vi "autoshoot.vi"() -> ()   [LabVIEW 2012]
uses:
  <vilib>/Platform/TimedLoop/XDataNode/wakeup.ctl
  <vilib>/Platform/TimedLoop/XDataNode/XDNodeRunTimeDep.lvlib
  <vilib>/Platform/TimedLoop/XDataNode/nitl_modes.ctl
  <vilib>/Platform/TimedLoop/XDataNode/timing_clust.ctl
  <vilib>/platform/TimedLoop/XDataNode/XDataNode.xnode
  <vilib>/Rock Robotics/WPI/RobotDrive/WPI_RobotDriveArcadeDrive_Standard(NoSaturation).vi
  <vilib>/Rock Robotics/WPI/Solenoid/WPI_SolenoidValue.ctl
  <vilib>/Rock Robotics/WPI/Solenoid/WPI_SolenoidSetEnum.vi
panel:
  out "seconds":dbl
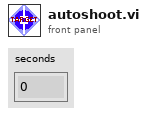
[diagram p1: front panel]
types:
  T1 = typedef "XDNodeRunTimeDep.lvlib/timing_clust.ctl" = cluster{"Expected End [f-1]":u64, "Actual End [f-1]":u64, "Finished Late? [f-1]":bool, "Expected End [i-1]":u64, "Actual End [i-1]":u64, "Finished Late? [i-1]":bool, "Expected Start [i]":u64, "Actual Start [i]":u64, "Expected Start [f]":u64, "Actual Start [f]":u64, "Source Name":string, "Structure Name":string, "Period":i64, "Deadline":i64, "Offset":i64, "Start":i64, "Priority":i32, "Timeout":i32, "Mode":T2, "Wakeup Reason":T3, "Error":errorcluster, "Source Type":string, "Secondary Source Type":string, "Global End Time":u64, "Global Start Time":u64, "Frame Duration":u64, "Iteration Duration":u64, "Assigned CPU":i32, "I/O Scan Engine Mode":u32}
  T2 = typedef "XDNodeRunTimeDep.lvlib/nitl_modes.ctl" = enum32{"No Change", "Process missed periods, maintain original phase", "Discard missed periods, maintain original phase", "Process missed periods, ignore original phase", "Discard missed periods, ignore original phase"}
  T3 = typedef "XDNodeRunTimeDep.lvlib/wakeup.ctl" = enum32{"Normal", "Aborted", "Asynchronous wakeup", "Timing source error", "Timed loop error", "Timeout"}
  T4 = typedef "WPI_SolenoidValue.ctl" = enum16{"Off", "On", "Forward", "Reverse"}
  T5 = typedef "WPI_AnalogChannelDevRef.ctl" = cluster{"DevStatus":errorcluster, "Analog Module":T6, "Analog Channel":T7}
  T6 = typedef "FPGA_TypedefAnalogModule.ctl" = enum16{"Analog Module 1", "Analog Module 2"}
  T7 = typedef "FPGA_AIChannel.ctl" = enum8{"AI 1", "AI 2", "AI 3", "AI 4", "AI 5", "AI 6", "AI 7", "AI 8", "Invalid"}
  T8 = typedef "WPI_RobotDriveDevRef.ctl" = cluster{"DevStatus":errorcluster, "Motors[]":T9[], "Square Inputs":bool, "Max Output":dbl, "Isochronous":bool}
  T9 = typedef "WPI_MotorControlDeviceRef.ctl" = cluster{"DeviceStatus":errorcluster, "Type":enum16{"PWM", "CAN"}, "PWM":cluster{"Digital Module":T10, "PWM Channel":T11, "DeadBand":T12}, "CAN":cluster{"Device Number":u8, "Control Mode":T13, "Semaphore":T14, "Max Vout":dbl}, "Invert":bool, "TransformRef":T15, "InvTransformRef":T15}
  T10 = typedef "FPGA_TypedefDigitalModule.ctl" = enum16{"Digital Module 1", "Digital Module 2"}
  T11 = typedef "FPGA_DIOPWMChannel.ctl" = enum8{"PWM 1", "PWM 2", "PWM 3", "PWM 4", "PWM 5", "PWM 6", "PWM 7", "PWM 8", "PWM 9", "PWM 10", "Invalid"}
  T12 = typedef "WPI_PWMDeadband.ctl" = cluster{"Name":string, "maxPositivePwm":i32, "minPositivePwm":i32, "centerPwm":i32, "maxNegativePwm":i32, "minNegativePwm":i32, "angularRange":u16}
  T13 = typedef "WPI_CANJaguar_ControlMode.ctl" = enum8{"Percent VBus", "Current", "Speed", "Position", "Voltage"}
  T14 = typedef "Semaphore RefNum" = refnum<k1>
  T15 = typedef "WPI_PWMTransform_ConPane.ctl" = refnum<vi>
  T16 = typedef "WPI_SolenoidDevRef.ctl" = cluster{"DevStatus":errorcluster, "Solenoid Module":T17, "Forward Solenoid Channel":T18, "Reverse Solenoid Channel":T18}
  T17 = typedef "FPGA_TypedefSolenoidModule.ctl" = enum16{"Solenoid Module 1", "Solenoid Module 2"}
  T18 = typedef "WPI_SolenoidChannel.ctl" = enum8{"Solenoid 1", "Solenoid 2", "Solenoid 3", "Solenoid 4", "Solenoid 5", "Solenoid 6", "Solenoid 7", "Solenoid 8", "Invalid"}
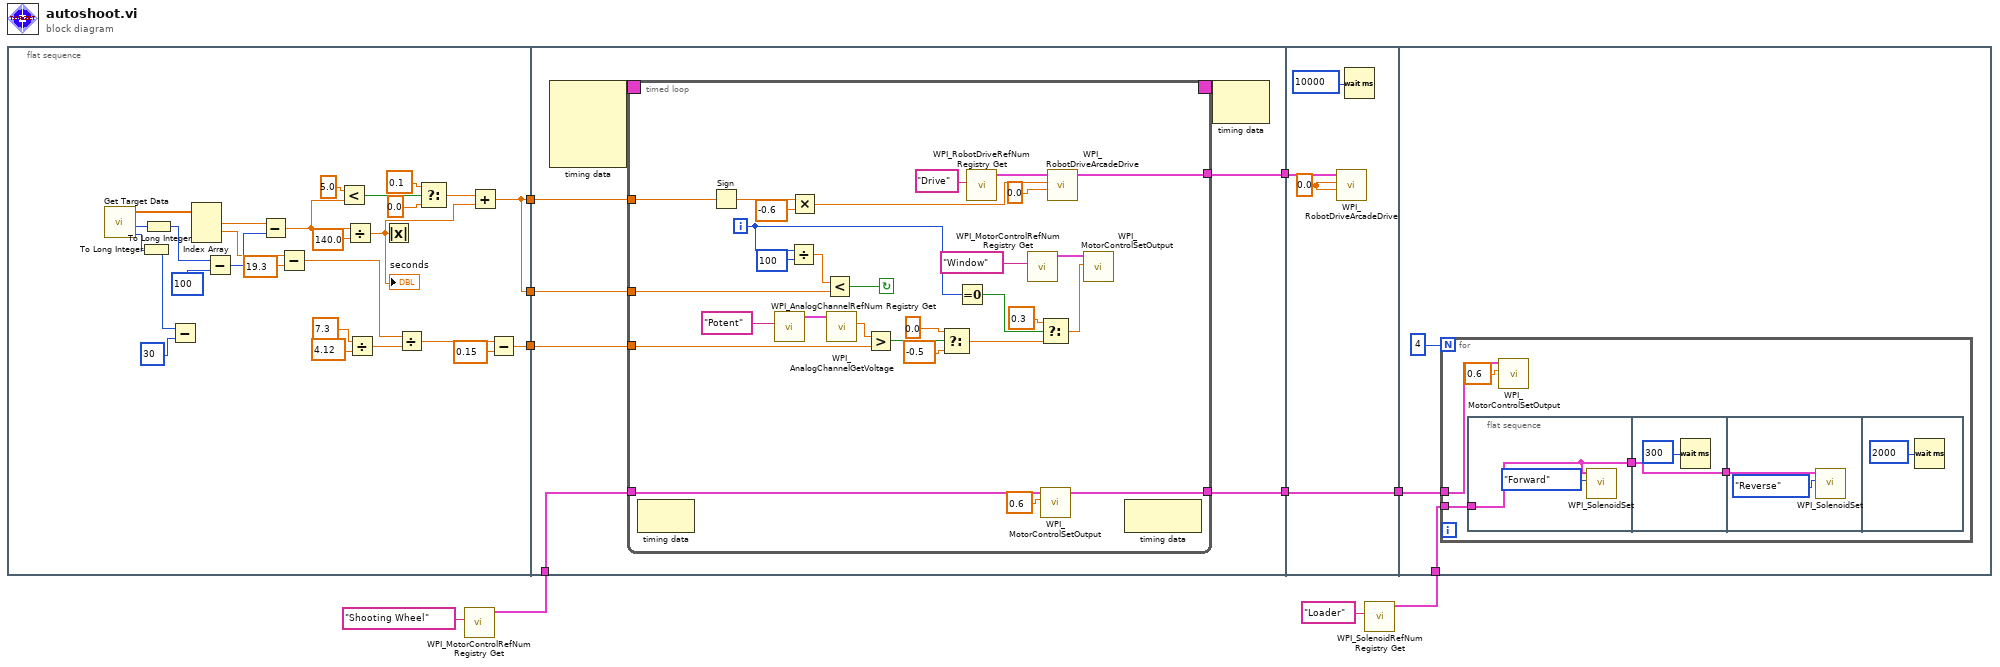
[diagram p0: block diagram]
diagram:
  n1 = flat-sequence {
    tunnel: [w29] -> w10
    tunnel: [w29] -> w9
    tunnel: [w14] -> w8
    tunnel: [w45] -> w7
    tunnel: w2 -> [w42]
    tunnel: w10 -> [w41]
    tunnel: w9 -> [w40]
    tunnel: [w39] -> w6
    tunnel: w8 -> [w38]
    tunnel: w7 -> [w82]
    tunnel: [w82] -> w5
    tunnel: w6 -> [w79]
    tunnel: w4 -> [w84]
    tunnel: w5 -> [w83]
    frame #0 {
      n2 = call "Get Target Data.vi"() -> ("y angle"=w13:u16, "x angle"=w32:u16, "Yellow"=w36:dbl[])  [unwired: 9 in]
      n3 = To Long Integer(number=w13) -> (32bit integer=w12:i32)
      n4 = To Long Integer(number=w32) -> (32bit integer=w33:i32)
      n5 = Subtract(x=w12, y=30) -> ()  [unwired: 1 out]
      n6 = Index Array(array=w36) -> (element #1=w34:dbl, element #2=w23:dbl)  [unwired: 3 in, 1 out]
      n7 = Subtract(x=w33, y=100) -> (x-y=w35:i32)
      n8 = Subtract(x=w34, y=w35) -> (x-y=w24:dbl)
      n9 = Subtract(x=w23, y=19.3) -> (x-y=w20:dbl)
      n10 = Less?(x=5.0, y=w24) -> (x < y?=w25:bool)
      n11 = Divide(x=w24, y=140.0) -> (x/y=w30:dbl)
      "seconds" <- w30
      n12 = Divide(x=7.3, y=4.12) -> (x/y=w19:dbl)
      n13 = Absolute Value(x=w30) -> ()  [unwired: 1 out]
      n14 = Divide(x=w20, y=w19) -> (x/y=w16:dbl)
      n15 = Select(t=0.1 ("x"), s=w25, f=0.0) -> (s? t:f=w27:dbl)
      n16 = Add(x=w27, y=w30) -> (x+y=w29:dbl)
      n17 = Subtract(x=w16, y=0.15) -> (x-y=w14:dbl)
    }
    frame #1 {
      n18 = node-c288() -> (w44:T1)  [unwired: 4 in]
      n19 = timed-loop {
        timing: w44 -> [_]
        timing-out: [_] -> w43
        tunnel: [w69] -> w45
        tunnel: w42 -> [w71]
        tunnel: w41 -> [w68]
        tunnel: w40 -> [w70]
        tunnel: [w61] -> w39
        tunnel: w38 -> [w51]
        i -> [w60]
        stop <- w74 continue-if-true
        n20 = node-c288() -> ()  [unwired: 1 in, 1 out]
        n21 = Sign(1:w68) -> (0:w67:dbl)
        n22 = call <vilib>:"WPI_AnalogChannelRefNum Registry Get.vi"("refnum name"="Potent") -> ("AIDeviceRef"=w52:T5)  [unwired: 9 in, 1 out]
        n23 = Divide(x=w60, y=100) -> (x/y=w72:dbl)
        n24 = Multiply(x=w67, y=-0.6) -> (x*y=w64:dbl)
        n25 = Less?(x=w72, y=w70) -> (x < y?=w74:bool)
        n26 = call <vilib>:"WPI_AnalogChannelGetVoltage.vi"("AIDeviceRef"=w52) -> ("Voltage"=w50:dbl)  [unwired: 8 in, 2 out]
        n27 = Greater?(x=w50, y=w51) -> (0:w49:bool)
        n28 = Select(t=0.0, s=w49, f=-0.5) -> (s? t:f=w46:dbl)
        n29 = Equal To 0?(x=w60) -> (x = 0?=w57:bool)
        n30 = call <vilib>:"WPI_RobotDriveRefNum Registry Get.vi"("refnum name"="Drive") -> ("RobotDriveDevRef"=w65:T8)  [unwired: 9 in, 1 out]
        n31 = call <vilib>:"WPI_MotorControlRefNum Registry Get.vi"("refnum name"="Window") -> ("MotorControlDevRef"=w58:T9)  [unwired: 9 in, 1 out]
        n32 = Select(t=0.3, s=w57, f=w46) -> (s? t:f=w56:dbl)
        n33 = call <vilib>:"WPI_MotorControlSetOutput.vi"("Output"=0.6, "MotorControlDevRef"=w71) -> ("MotorControlDevRef"=w69:T9)  [unwired: 7 in, 2 out]
        n34 = call-poly <vilib>:"WPI_RobotDriveArcadeDrive.vi"("Y axis value"=0.0, "X axis value"=w64, "RobotDriveDevRef"=w65) -> ("RobotDriveDevRef"=w61:T8)  [unwired: 6 in, 2 out]
        n35 = call <vilib>:"WPI_MotorControlSetOutput.vi"("Output"=w56, "MotorControlDevRef"=w58) -> ()  [unwired: 7 in, 3 out]
        n36 = node-c288() -> ()  [unwired: 1 in, 1 out]
      }
      n37 = node-c288(w43) -> ()  [unwired: 1 out]
    }
    frame #2 {
      w80 = 0.0 ("X axis value")
      n38 = call-poly <vilib>:"WPI_RobotDriveArcadeDrive.vi"("Y axis value"=w80, "X axis value"=w80, "RobotDriveDevRef"=w79) -> ()  [unwired: 6 in, 3 out]
      n39 = Wait (ms)(milliseconds to wait=u32 10000) -> ()  [unwired: 1 out]
    }
    frame #3 {
      n40 = for {
        N: 4 -> [_]
        tunnel: w84 -> [w90]
        tunnel: w83 -> [w87]
        n41 = flat-sequence {
          tunnel: w90 -> [w91]
          tunnel: [w91] -> w89
          tunnel: w89 -> [w94]
          tunnel: [w94] -> w88
          tunnel: w88 -> [w95]
          frame #0 {
            n42 = call-poly <vilib>:"WPI_SolenoidSet.vi"("Value"=WPI_SolenoidValue."Forward", "SolenoidDevRef"=w91) -> ()  [unwired: 8 in, 2 out]
          }
          frame #1 {
            n43 = Wait (ms)(milliseconds to wait=u32 300) -> ()  [unwired: 1 out]
          }
          frame #2 {
            n44 = call-poly <vilib>:"WPI_SolenoidSet.vi"("Value"=WPI_SolenoidValue."Reverse", "SolenoidDevRef"=w95) -> ()  [unwired: 8 in, 2 out]
          }
          frame #3 {
            n45 = Wait (ms)(milliseconds to wait=u32 2000) -> ()  [unwired: 1 out]
          }
        }
        n46 = call <vilib>:"WPI_MotorControlSetOutput.vi"("Output"=0.6, "MotorControlDevRef"=w87) -> ()  [unwired: 7 in, 3 out]
      }
    }
  }
  n47 = call <vilib>:"WPI_MotorControlRefNum Registry Get.vi"("refnum name"="Shooting Wheel") -> ("MotorControlDevRef"=w2:T9)  [unwired: 9 in, 1 out]
  n48 = call <vilib>:"WPI_SolenoidRefNum Registry Get.vi"("refnum name"="Loader") -> ("SolenoidDevRef"=w4:T16)  [unwired: 9 in, 1 out]
